vi "Noise Bandwidth for Cascaded 1st Order Filter.vi"(10 "b[i]":dbl[](array[numeric]) format="%.2f", 11 "a[i]":dbl[](array[numeric]) format="%.2f") -> (2 "noise bandwidth":dbl format="%#.6g")   [LabVIEW 2020, in "NI_AALBase.lvlib"]
uses:
  <vilib>/Analysis/NI_AALBase.lvlib
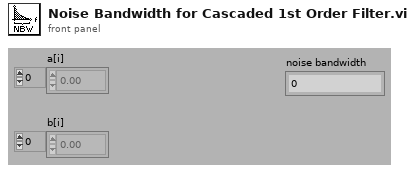
[diagram p1: front panel]
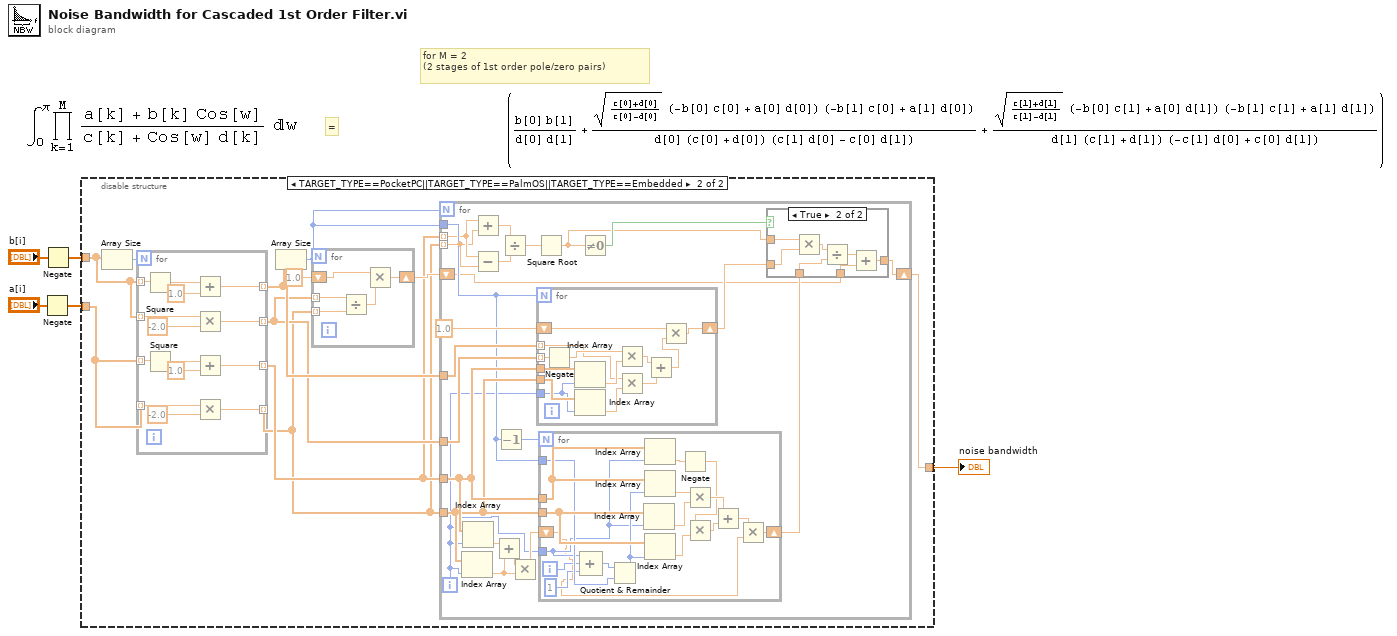
[diagram p0: block diagram]
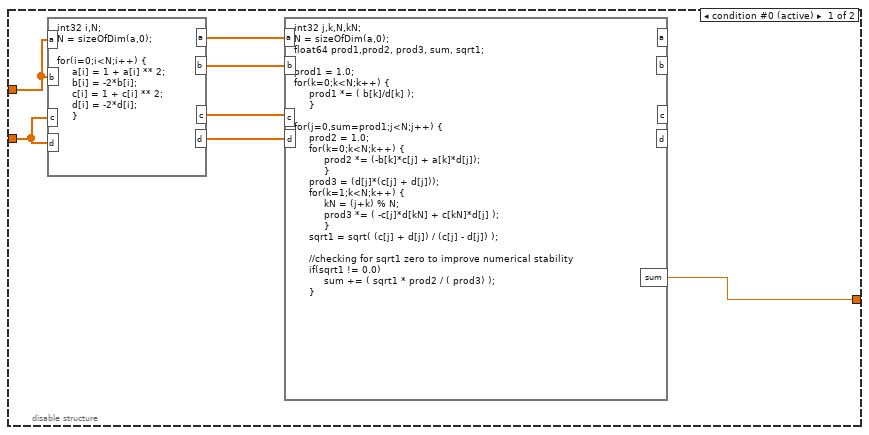
[diagram p2: hidden frame]
diagram:
  # "for M = 2 \n(2 stages of 1st order pole/zero pairs)"
  # "="
  n1 = Negate(x="a[i]") -> (-x=w2:dbl[])
  n2 = Negate(x="b[i]") -> (-x=w3:dbl[])
  n3 = disable-structure shown="TARGET_TYPE==PocketPC||TARGET_TYPE==PalmOS||TARGET_TYPE==Embedded" {
    disable-tunnel: w3 -> [w8 w22]
    disable-tunnel: w2 -> [w7 w21]
    disable-tunnel: [w6 w13] -> w1
    frame condition #0 (active) {
      n4 = formula code="int32 i,N;\nN = sizeOfDim(a,0);\n\nfor(i=0;i<N;i++) {\n     a[i] = 1 + a[i] ** 2;\n     b[i] = -2*b[i];\n     c[i] = 1 + c[i] ** 2;\n     d[i] = -2*d[i];\n     }"("a"=w8, "b"=w8, "c"=w7, "d"=w7) -> ("a"=w12:dbl[], "b"=w11:dbl[], "c"=w10:dbl[], "d"=w9:dbl[])
      n5 = formula code="int32 j,k,N,kN;\nN = sizeOfDim(a,0);\nfloat64 prod1,prod2, prod3, sum, sqrt1;\n\nprod1 = 1.0;\nfor(k=0;k<N;k++) {\n     prod1 *= ( b[k]/d[k] );\n     }\n\nfor(j=0,sum=prod1;j<N;j++) {\n     prod2 = 1.0;\n     for(k=0;k<N;k++) {\n          prod2 *= (-b[k]*c[j] + a[k]*d[j]);\n          }\n     prod3 = (d[j]*(c[j] + d[j]));\n     for(k=1;k<N;k++) {\n          kN = (j+k) % N;\n          prod3 *= ( -c[j]*d[kN] + c[kN]*d[j] );\n          }\n     sqrt1 = sqrt( (c[j] + d[j]) / (c[j] - d[j]) );\n\n     //checking for sqrt1 zero to improve numerical stability\n     if(sqrt1 != 0.0)\n          sum += ( sqrt1 * prod2 / ( prod3) );\n     }"("a"=w12, "b"=w11, "c"=w10, "d"=w9) -> ("sum"=w6:dbl)  [unwired: 4 out]
    }
    frame condition #1 {
      n6 = Array Size(array=w22) -> (size(s)=w23:i32)
      n7 = for {
        N: w23 -> [_]
        tunnel: w22 -> [w96] mode=indexing
        tunnel: w22 -> [w101] mode=indexing
        tunnel: w21 -> [w98] mode=indexing
        tunnel: w21 -> [w104] mode=indexing
        tunnel: [w102] -> w14 mode=indexing
        tunnel: [w99] -> w17 mode=indexing
        tunnel: [w92] -> w15 mode=indexing
        tunnel: [w91] -> w18 mode=indexing
        n8 = Square(x=w96) -> (x^2=w95:dbl)
        n9 = Square(x=w98) -> (x^2=w97:dbl)
        n10 = Add(x=w95, y=1.0) -> (x+y=w91:dbl)
        n11 = Multiply(x=w101, y=-2.0) -> (x*y=w99:dbl)
        n12 = Add(x=w97, y=1.0) -> (x+y=w92:dbl)
        n13 = Multiply(x=w104, y=-2.0) -> (x*y=w102:dbl)
      }
      n14 = Array Size(array=w18) -> (size(s)=w16:i32)
      n15 = for {
        N: w16 -> [_]
        tunnel: w17 -> [w89] mode=indexing
        tunnel: w14 -> [w90] mode=indexing
        shift-right: [w87] -> w19
        shift-left: 1.0 -> [w86]
        n16 = Divide(x=w89, y=w90) -> (x/y=w88:dbl)
        n17 = Multiply(x=w86, y=w88) -> (x*y=w87:dbl)
      }
      n18 = for {
        N: w16 -> [_]
        tunnel: w18 -> [w45]
        tunnel: w17 -> [w44]
        tunnel: w15 -> [w43]
        tunnel: w14 -> [w42]
        tunnel: w16 -> [w36]
        tunnel: w15 -> [w32] mode=indexing
        tunnel: w14 -> [w31] mode=indexing
        shift-right: [w28] -> w13
        shift-left: w19 -> [w24]
        i -> [w35]
        n19 = Index Array(array=w42, index=w35) -> (element=w39:dbl)
        n20 = Index Array(array=w43, index=w35) -> (element=w40:dbl)
        n21 = Add(x=w32, y=w31) -> (x+y=w33:dbl)
        n22 = Subtract(x=w32, y=w31) -> (x-y=w34:dbl)
        n23 = Add(x=w40, y=w39) -> (x+y=w38:dbl)
        n24 = Decrement(x=w36) -> (x-1=w37:i32)
        n25 = Divide(x=w33, y=w34) -> (x/y=w30:dbl)
        n26 = Multiply(x=w38, y=w39) -> (x*y=w41:dbl)
        n27 = Square Root(x=w30) -> (sqrt(x)=w26:dbl)
        n28 = for {
          N: w36 -> [_]
          shift-right: [w85] -> w25
          shift-left: 1.0 -> [w84]
          tunnel: w45 -> [w74] mode=indexing
          tunnel: w44 -> [w83] mode=indexing
          tunnel: w43 -> [w82]
          tunnel: w42 -> [w81]
          tunnel: w35 -> [w80]
          n29 = Negate(x=w83) -> (-x=w76:dbl)
          n30 = Index Array(array=w82, index=w80) -> (element=w75:dbl)
          n31 = Index Array(array=w81, index=w80) -> (element=w73:dbl)
          n32 = Multiply(x=w76, y=w75) -> (x*y=w79:dbl)
          n33 = Multiply(x=w74, y=w73) -> (x*y=w78:dbl)
          n34 = Add(x=w79, y=w78) -> (x+y=w77:dbl)
          n35 = Multiply(x=w84, y=w77) -> (x*y=w85:dbl)
        }
        n36 = for {
          N: w37 -> [_]
          tunnel: w43 -> [w72]
          tunnel: w42 -> [w71]
          shift-right: [w58] -> w27
          shift-left: w41 -> [w56]
          tunnel: w35 -> [w65]
          tunnel: w36 -> [w70]
          i -> [w67]
          n37 = Compound Arithmetic op=ADD(w65, w67, 1 ("value")) -> (w69:i32)
          n38 = Quotient & Remainder(x=w69, y=w70) -> (x-y*floor(x/y)=w66:i32)  [unwired: 1 out]
          n39 = Index Array(array=w71, index=w65) -> (element=w63:dbl)
          n40 = Index Array(array=w72, index=w65) -> (element=w62:dbl)
          n41 = Index Array(array=w72, index=w66) -> (element=w64:dbl)
          n42 = Index Array(array=w71, index=w66) -> (element=w61:dbl)
          n43 = Negate(x=w62) -> (-x=w55:dbl)
          n44 = Multiply(x=w64, y=w63) -> (x*y=w59:dbl)
          n45 = Multiply(x=w55, y=w61) -> (x*y=w60:dbl)
          n46 = Add(x=w59, y=w60) -> (x+y=w57:dbl)
          n47 = Multiply(x=w57, y=w56) -> (x*y=w58:dbl)
        }
        n48 = Not Equal To 0?(x=w26) -> (x != 0?=w29:bool)
        n49 = case shown="True" w29 {
          tunnel: [w47 w50] -> w28
          tunnel: w27 -> [_ w52]
          tunnel: w26 -> [_ w54]
          tunnel: w25 -> [_ w53]
          tunnel: w24 -> [w47 w49]
          frame False {
          }
          frame True {
            n50 = Multiply(x=w54, y=w53) -> (x*y=w51:dbl)
            n51 = Divide(x=w51, y=w52) -> (x/y=w48:dbl)
            n52 = Add(x=w48, y=w49) -> (x+y=w50:dbl)
          }
        }
      }
    }
  }
  "noise bandwidth" <- w1
